vi "Get Control Size.vi"(7 "CtrlRef":refnum<vi>) -> (8 "Size":T1)   [LabVIEW 2011]
uses:
  <vilib>/Utility/miscctls.llb/LVBoundsTypeDef.ctl
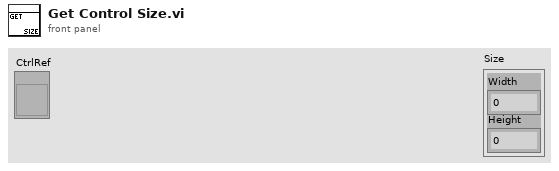
[diagram p1: front panel]
types:
  T1 = typedef "LVBoundsTypeDef.ctl" = cluster{"Width":u32, "Height":u32}
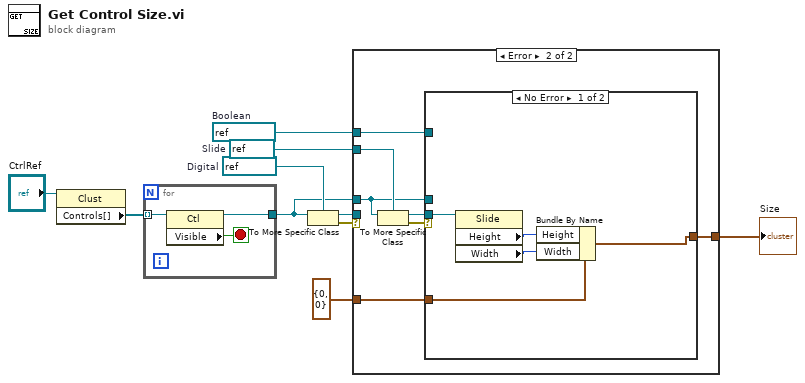
[diagram p0: block diagram]
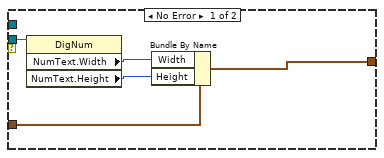
[diagram p2: hidden frame]
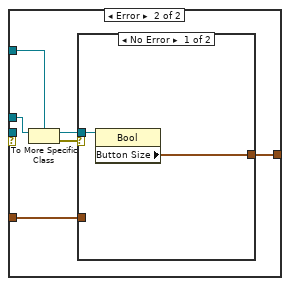
[diagram p3: hidden frame]
diagram:
  w4 = refnum<vi> refnum  # Boolean
  w5 = refnum<vi> refnum  # Slide
  w9 = refnum<vi> refnum  # Digital
  n1 = property class="Clust"(reference="CtrlRef") -> ("Controls[]"=w10:refnum<vi>[])  [unwired: 1 in, 2 out]
  n2 = for {
    tunnel: w10 -> [w13] mode=indexing
    tunnel: [w11] -> w1
    stop <- w12 stop-if-true
    n3 = property class="Ctl"(reference=w13) -> (reference out=w11:refnum<vi>, "Visible"=w12:bool)  [unwired: 1 in, 1 out]
  }
  n4 = To More Specific Class(target class=w9, reference=w1) -> (specific class reference=w6:refnum<vi>, error out=w7:errorcluster)  [unwired: 1 in]
  n5 = case shown="Error" w7 {
    tunnel: w6 -> [w18 _]
    tunnel: w5 -> [_ w25]
    tunnel: w4 -> [_ w22]
    tunnel: T1 {"Width"=0, "Height"=0} ("Size") -> [w17 w21]
    tunnel: [w15 w20] -> w2
    tunnel: w1 -> [_ w19]
    frame No Error {
      n6 = property class="DigNum"(reference=w18) -> ("NumText.Width"=w16:u32, "NumText.Height"=w14:u32)  [unwired: 1 in, 2 out]
      n7 = Bundle By Name(cluster=w17, "Width"=w16, "Height"=w14) -> (w15:T1)
    }
    frame Error {
      n8 = To More Specific Class(target class=w25, reference=w19) -> (specific class reference=w24:refnum<vi>, error out=w23:errorcluster)  [unwired: 1 in]
      n9 = case shown="No Error" w23 {
        tunnel: w24 -> [w30 _]
        tunnel: w22 -> [_ w36]
        tunnel: w21 -> [w29 w32]
        tunnel: [w28 w33] -> w20
        tunnel: w19 -> [_ w31]
        frame No Error {
          n10 = property class="Slide"(reference=w30) -> ("Height"=w27:u32, "Width"=w26:u32)  [unwired: 1 in, 2 out]
          n11 = Bundle By Name(cluster=w29, "Height"=w27, "Width"=w26) -> (w28:T1)
        }
        frame Error {
          n12 = To More Specific Class(target class=w36, reference=w31) -> (specific class reference=w34:refnum<vi>, error out=w35:errorcluster)  [unwired: 1 in]
          n13 = case shown="No Error" w35 {
            tunnel: w34 -> [w38 _]
            tunnel: [w37 w39] -> w33
            tunnel: w32 -> [_ w39]
            frame No Error {
              n14 = property class="Bool"(reference=w38) -> ("Button Size"=w37:T1)  [unwired: 1 in, 2 out]
            }
            frame Error {
            }
          }
        }
      }
    }
  }
  "Size" <- w2
